vi "Update Analysis 3D U16.vi"(8 "error in (no error)":errorcluster, 9 "Image Series":u16[][][](array[numeric]), 10 "Analysis Image":dbl[][](array[numeric]), 11 "Analysis Graph in":refnum<class "Analysis Graph.lvclass">) -> (0 "error out":errorcluster, 1 "pixel signal roied  out":u16[](array[numeric]), 2 "Cursor.Cursor Position":T1, 3 "Analysis Graph out":refnum<class "Analysis Graph.lvclass">)   [LabVIEW 2023, in "Analysis Graph.lvclass"]
uses:
  Analysis Graph.lvclass
  <vilib>/Utility/miscctls.llb/LVPointDoubleTypeDef.ctl
  Series Graph/Series Graph.lvclass/Series Graph.ctl
  Analysis Graph.lvclass/Analysis Graph.ctl
  Detail Graph/Detail Graph.lvclass
  Series Graph/Series Graph.lvclass
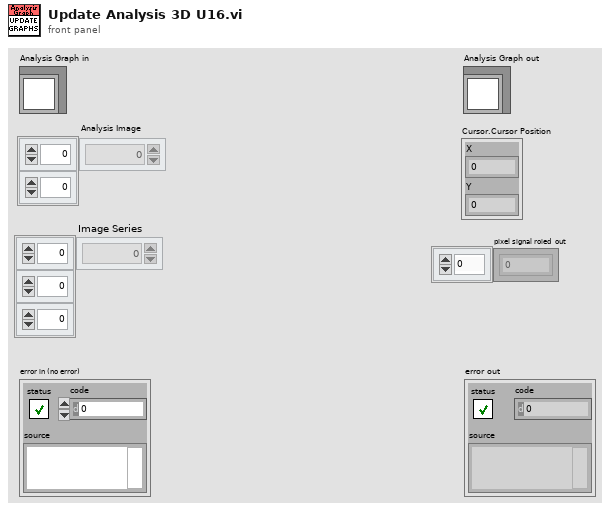
[diagram p1: front panel]
types:
  T1 = typedef "LVPointDoubleTypeDef.ctl" = cluster{"X":dbl, "Y":dbl}
  T2 = cluster{"ROI X":cluster{"Index":u32, "Length":u32}, "ROI Y":cluster{"Index":u32, "Length":u32}, "ROI Z":cluster{"Index":u32, "Length":u32}}
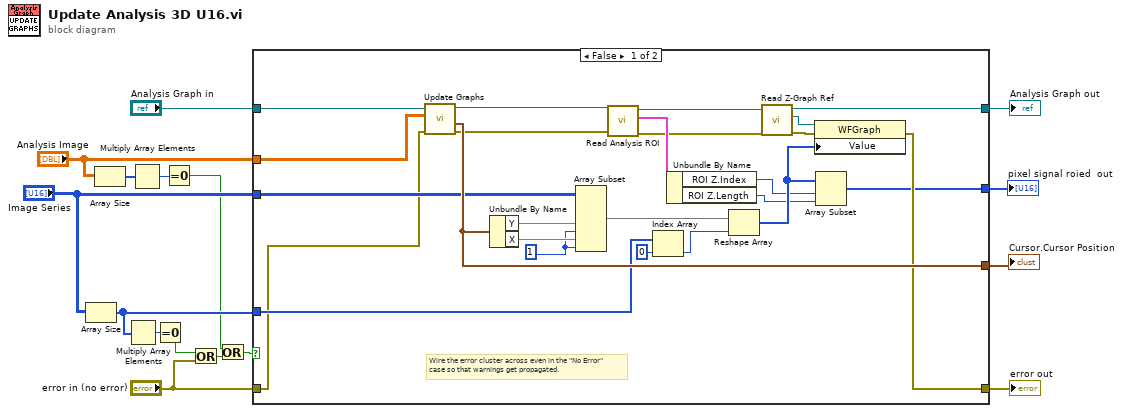
[diagram p0: block diagram]
diagram:
  n1 = Array Size(array="Image Series") -> (size(s)=w10:i32[])
  n2 = Array Size(array="Analysis Image") -> (size(s)=w5:i32[])
  n3 = Multiply Array Elements(1:w10) -> (0:w13:i32)
  n4 = Multiply Array Elements(1:w5) -> (0:w4:i32)
  n5 = Equal To 0?(x=w13) -> (x = 0?=w12:bool)
  n6 = Equal To 0?(x=w4) -> (x = 0?=w3:bool)
  n7 = Or(x=w12, y="error in (no error)") -> (x .or. y?=w2:bool)
  n8 = Or(x=w3, y=w2) -> (x .or. y?=w1:bool)
  n9 = case shown="False" w1 {
    tunnel: [w33 w42] -> w16
    tunnel: [w38 w43] -> w14
    tunnel: "Analysis Graph in" -> [w24 w43]
    tunnel: "error in (no error)" -> [w23 w42]
    tunnel: w10 -> [w29 _]
    tunnel: "Analysis Image" -> [w35 _]
    tunnel: "Image Series" -> [w32 _]
    tunnel: [w34 _] -> w8
    tunnel: [w17 _] -> w7
    frame False {
      w39 = 1 ("length")
      # "Wire the error cluster across even in the \"No Error\"\ncase so that warnings get propagated."
      n10 = call "Update Graphs.vi"("error in (no error)"=w23, "image"=w35, "Detail Graph in"=w24) -> ("error out"=w26:errorcluster, "Cursor.Cursor Position"=w34:T1, "Detail Graph out"=w22:refnum<class "Analysis Graph.lvclass">)  [unwired: 6 in]
      n11 = Unbundle By Name(w34) -> ("Y"=w41:dbl, "X"=w40:dbl)
      n12 = Array Subset(array=w32, index (dim 1)=w41, length (dim 1)=w39, index (dim 2)=w40, length (dim 2)=w39) -> (w28:u16[][][])  [unwired: 2 in]
      n13 = call "Read Analysis ROI.vi"("error in (no error)"=w26, "Analysis Graph in"=w22) -> ("error out"=w25:errorcluster, "ROI XYZ"=w27:T2, "Analysis Graph out"=w21:refnum<class "Analysis Graph.lvclass">)  [unwired: 7 in]
      n14 = Index Array(array=w29, index=0) -> (element=w31:i32)
      n15 = Unbundle By Name(w27) -> ("ROI Z.Index"=w19:u32, "ROI Z.Length"=w18:u32)
      n16 = Reshape Array(w28, w31) -> (w20:u16[])
      n17 = call "Read Z-Graph Ref.vi"("error in (no error)"=w25, "Series Graph in"=w21) -> ("error out"=w36:errorcluster, "Z-Graph Ref"=w37:refnum<vi>, "Series Graph out"=w38:refnum<class "Analysis Graph.lvclass">)  [unwired: 7 in]
      n18 = property class="WFGraph"(reference=w37, error in=w36, "Value"=w20) -> (error out=w33:errorcluster)  [unwired: 1 out]
      n19 = Array Subset(array=w20, index=w19, length=w18) -> (w17:u16[])
    }
    frame True {
    }
  }
  "error out" <- w16
  "Analysis Graph out" <- w14
  "Cursor.Cursor Position" <- w8
  "pixel signal roied  out" <- w7
